vi "Configure Output Timer.vi"(0 "VISA resource name":refnum<visa-resource-name>, 1 "Enable Timed Output (F: False)":bool, 5 "Timer Hour (0)":u32 max=99 step=1, 7 "Timer Minutes (0)":u32 max=59 step=1, 9 "Timer Seconds (0)":u32 max=59 step=1, 11 "error in (no error)":errorcluster) -> (4 "VISA resource name out":refnum<visa-resource-name>, 15 "error out":errorcluster)   [LabVIEW 2015, in "BK Precision 983X Series.lvlib"]
doc: "Configures the timer for timed output."
uses:
  <instrlib>/BK Precision 983X Series/BK Precision 983X Series.lvlib
panel:
  # "minutes"
  # "seconds"
  # "hours"
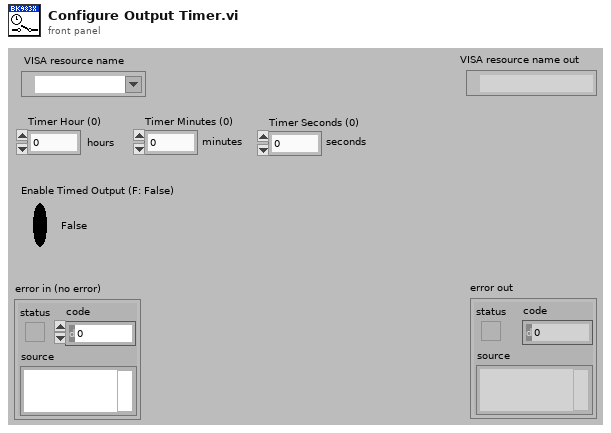
[diagram p1: front panel]
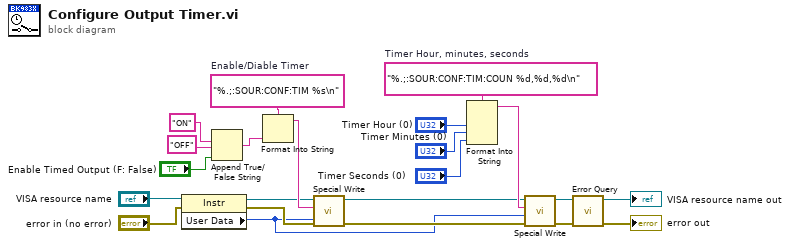
[diagram p0: block diagram]
diagram:
  w18 = "%.;:SOUR:CONF:TIM %s\n"  # Enable/Diable Timer
  w20 = "%.;:SOUR:CONF:TIM:COUN %d,%d,%d\n"  # Timer Hour, minutes, seconds
  n1 = property class="Instr"(reference="VISA resource name", error in="error in (no error)") -> (reference out=w7:refnum<visa-resource-name>, error out=w8:errorcluster, "User Data"=w1:u32)
  n2 = Append True/False String(1:"Enable Timed Output (F: False)", 2:"OFF" ("false string"), 3:"ON" ("true string")) -> (0:w12:string)  [unwired: 1 in]
  n3 = Format Into String(format string=w18, w12) -> (resulting string=w9:string)  [unwired: 2 in, 1 out]
  n4 = call <instrlib>:"Special Write.vi"("error in (no error)"=w8, "Delay (0 ms)"=w1, "Input String"=w9, "VISA resource name"=w7) -> ("error out"=w2:errorcluster, "VISA resource name out"=w3:refnum<visa-resource-name>)  [unwired: 6 in]
  n5 = Format Into String(format string=w20, "Timer Hour (0)", "Timer Minutes (0)", "Timer Seconds (0)") -> (resulting string=w4:string)  [unwired: 2 in, 1 out]
  n6 = call <instrlib>:"Special Write.vi"("error in (no error)"=w2, "Delay (0 ms)"=w1, "Input String"=w4, "VISA resource name"=w3) -> ("error out"=w5:errorcluster, "VISA resource name out"=w6:refnum<visa-resource-name>)  [unwired: 6 in]
  n7 = call <instrlib>:"Error Query.vi"("error in (no error)"=w5, "VISA resource name"=w6) -> ("error out"=→"error out":errorcluster, "VISA resource name out"=→"VISA resource name out":refnum<visa-resource-name>)  [unwired: 6 in, 2 out]
